vi "Global 40001 register.vi"() -> ()   [LabVIEW 2020]
panel:
  out "16 bit register - WORD":bool[](array[boolean])
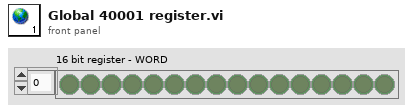
[diagram p1: front panel]
diagram:
